vi "global_exit.vi"() -> ()   [LabVIEW 2011, in "Fiberscope_library.lvlib"]
uses:
  Fiberscope_library.lvlib
panel:
  out "Global_exit":bool
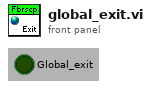
[diagram p1: front panel]
diagram:
